vi "PID Project.vi"() -> ()   [LabVIEW 2020]
uses:
  <vilib>/addons/control/pid/pid.llb/PID Advanced (DBL).vi
  <vilib>/addons/control/pid/NI_PID_pid.lvlib
panel:
  out "Liquid Control Value (LCV)":dbl(knob) scale=0.0..100.0
  out "Tank Process Output":dbl(slide) scale=0.0..100.0
  in  "Stop":bool
  out "Waveform Chart":T1(graph)
  in  "process parameters":T2={"static gain"=2.5, "lag (s)"=2.5, "deadtime (s)"=0.001, "load"=0.0, "deadband"=0.0, "sensor noise"=0.0, "initial PV"=30.0, "plant noise"=0.0} {"plant noise" format="%.2f"; "initial PV" format="%.2f"; "sensor noise" format="%.2f"; "lag (s)" format="%.2f"; "deadtime (s)" format="%.2f"; "deadband" format="%.1f"; "load" format="%.2f"; "static gain" format="%.2f"}
  in  "PID gains":T3={"proportional gain (Kc)"=1.0, "integral time (Ti, min)"=0.01, "derivative time (Td, min)"=0.0} {"derivative time (Td, min)" format="%.3f"; "integral time (Ti, min)" format="%.3f"; "proportional gain (Kc)" format="%.3f"}
  in  "Set Point":dbl(slide) scale=0.0..100.0
  in  "Auto Control":bool=TRUE
  in  "Manual Control":dbl format="%.2f"
  # "PID control of Liquid Tank"
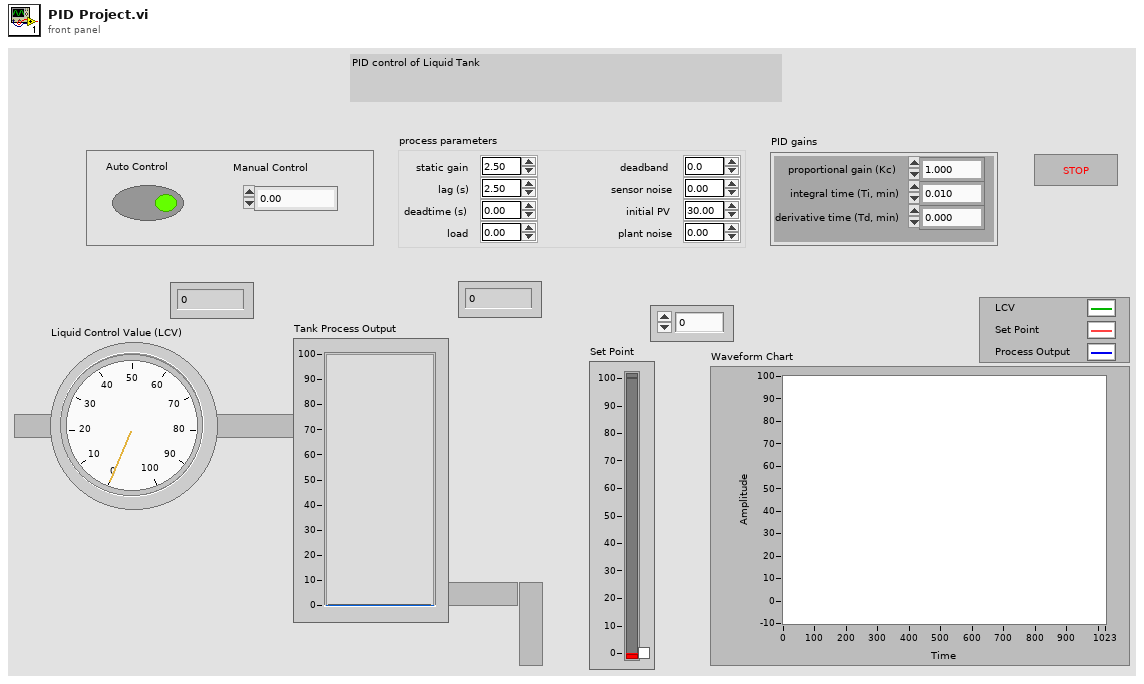
[diagram p1: front panel]
types:
  T1 = cluster{"Liquid Control Valve  (LCV)":dbl, "Set Point":dbl, "Plant Output":dbl}
  T2 = cluster{"static gain":dbl, "lag (s)":dbl, "deadtime (s)":dbl, "load":dbl, "deadband":dbl, "sensor noise":dbl, "initial PV":dbl, "plant noise":dbl}
  T3 = cluster{"proportional gain (Kc)":dbl, "integral time (Ti, min)":dbl, "derivative time (Td, min)":dbl}
  T4 = cluster{"output":dbl, "Set Point":dbl, "Plant Output":dbl}
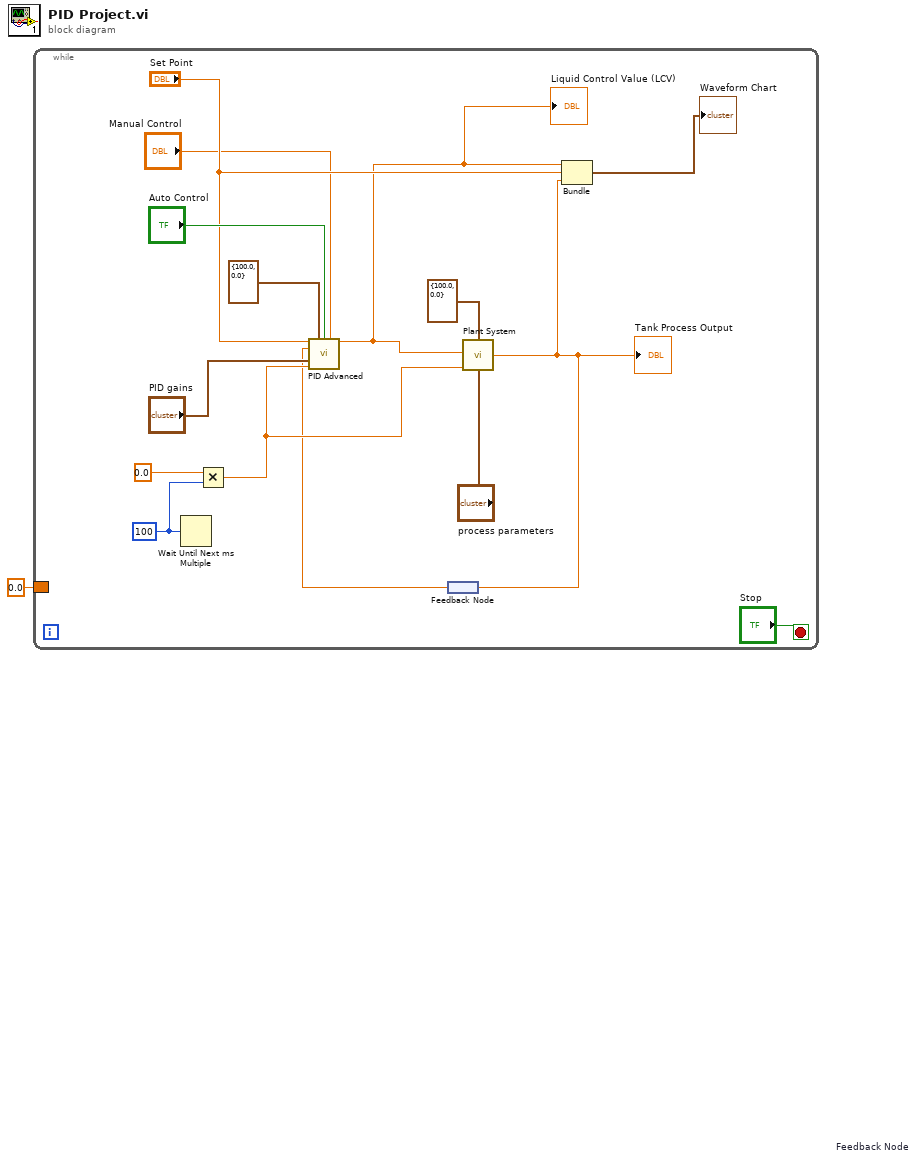
[diagram p0: block diagram]
diagram:
  n1 = while {
    border: 0.0 ("Plant Output") -> [_]
    stop <- "Stop" stop-if-true
    w12 = u32 100 ("millisecond multiple")
    n2 = Wait Until Next ms Multiple(millisecond multiple=w12) -> ()  [unwired: 1 out]
    n3 = Multiply(x=0.0, y=w12) -> (x*y=w11:dbl)
    n4 = feedback #1 "Feedback Node"() -> (w8:dbl)
    n5 = call-poly <vilib>:"PID Advanced.vi"("setpoint"="Set Point", "output range"=cluster{"output high":dbl, "output low":dbl} {"output high"=100.0, "output low"=0.0}, "auto? (T)"="Auto Control", "manual control"="Manual Control", "process variable"=w8, "PID gains"="PID gains", "dt (s)"=w11) -> ("output"=w2:dbl)  [unwired: 7 in, 1 out]
    "Liquid Control Value (LCV)" <- w2
    n6 = call "Plant System.vi"("output saturation range"=cluster{"output high":dbl, "output low":dbl} {"output high"=100.0, "output low"=0.0}, "Plant Input"=w2, "dt (s)"=w11, "process parameters"="process parameters") -> ("Plant Output"=w7:dbl)  [unwired: 11 in]
    "Tank Process Output" <- w7
    n7 = feedback-in #1(w7) -> ()
    n8 = Bundle("output"=w2, "Set Point"="Set Point", "Plant Output"=w7) -> (→"Waveform Chart":T4)  [unwired: 1 in]
  }
